vi "find_custom.vi"(8 "error in (no error)":errorcluster, 9 "find_custom params":T1, 10 "Field of View":T2, 11 "Image":T3) -> (0 "error out":errorcluster, 3 "Found Points":cluster{"x":dbl, "y":dbl}[](array[cluster]))   [LabVIEW 2024, in "Vision.lvlib"]
uses:
  Vision.lvlib
  <vilib>/vision/Image Controls.llb/IMAQ Image.ctl
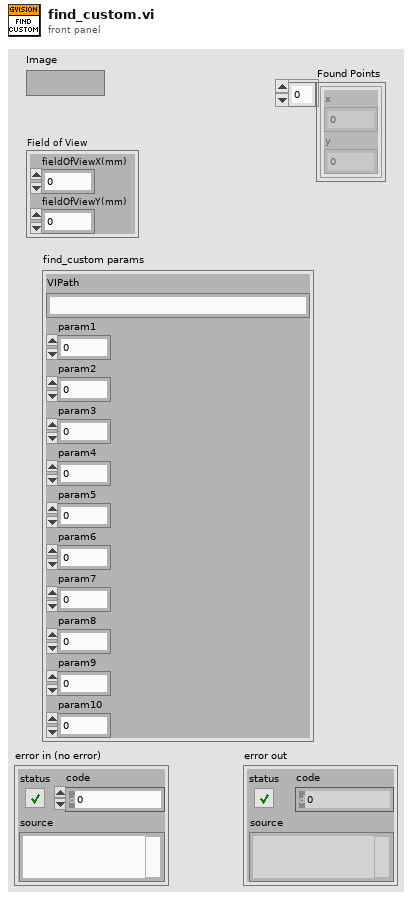
[diagram p1: front panel]
types:
  T1 = cluster{"VIPath":string, "param1":dbl, "param2":dbl, "param3":dbl, "param4":dbl, "param5":dbl, "param6":dbl, "param7":dbl, "param8":dbl, "param9":dbl, "param10":dbl}
  T2 = cluster{"fieldOfViewX(mm)":sgl, "fieldOfViewY(mm)":sgl}
  T3 = typedef "IMAQ Image.ctl" = refnum<image>
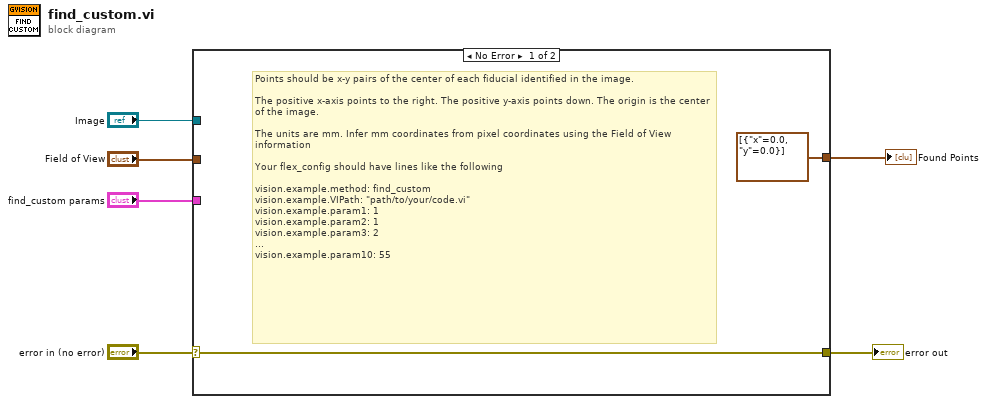
[diagram p0: block diagram]
diagram:
  n1 = case shown="No Error" "error in (no error)" {
    selector: "error in (no error)" -> [w8 w9]
    tunnel: [w8 w9] -> w5
    tunnel: "Image" -> [_ _]
    tunnel: "Field of View" -> [_ _]
    tunnel: [cluster{"x":dbl, "y":dbl}[] [{"x"=0.0, "y"=0.0}] ("Found Points 2") _] -> w2
    tunnel: "find_custom params" -> [_ _]
    frame No Error {
      # "Points should be x-y pairs of the center of each fiducial identified in the image. \n\nThe positive x-axis points to the right. The positive y-axis points down. The origin is the center of the image.\n\nThe units are mm. Infer mm coordinates from pixel coordinates using the Field of View information\n\nYour flex_config should have lines like the following\n\nvision.example.method: find_custom\nvision.example.VIPath: \"path/to/your/code.vi\"\nvision.example.param1: 1\nvision.example.param2: 1\nvision.example.param3: 2\n...\nvision.example.param10: 55"
    }
    frame Error {
    }
  }
  "error out" <- w5
  "Found Points" <- w2
